vi "ni579x Configure Output Power.vi"(0 "Register Bus":T1, 1 "scope":string="tx", 5 "output power [dBm]":dbl, 9 "frequency [Hz]":dbl format="%#_6p", 11 "Error In":errorcluster, 12 "characterization data":T2 {"Frequencies [Hz]" format="%#_6p"}, 13 "correct IQ imbalance?":bool=TRUE) -> (4 "Register Bus (out)":T1, 6 "coerced output power [dBm]":dbl, 8 "digital gain":T6, 10 "IQ impairment correction":T5, 15 "Error Out":errorcluster)   [LabVIEW 2015, in "ni579x Config v2 Host.lvlib"]
doc: "Configures the Tx front end attenuators and filters to achieve the specified output power, returns the IQ impairment correction data which can be used to correct IQ impairments, and returns the residual digital gain that can be applied to the signal to achieve the specified output power. Also sets the RF filter appropriately for the specified frequency.\n\n<B>Input Parameters</B>\n\n<B>Register Bus</B> The Register Bus object created by the ni579x Open VI and used as the session handle for the NI-579x Configuration Design Library.\n\n<B>scope</B> Specifies which channel to configure. Can be \"tx\".\n\n<B>output power [dBm]</B> Specifies the power (in dBm) at the output terminal of the device that will correspond to the full-scale range of the DAC binary data.\n\n<B>frequency [Hz]</B> Specifies the frequency the LO is tuned to in the current configuration.\n\n<B>correct IQ imbalance?</B> Specifies whether this VI should calculate the IQ impairment correction values. Set to false if you are not using the IQ impairment correction DSP blocks in the FPGA.\n\n<B>characterization data</B> A set of data that describes the characteristics of this device that allows the VI to calculate the proper attenuation and IQ imbalance correction settings for the specified frequency. This data is stored in the EEPROM and can be retrieved using the ni579x Load Characterization Data (EEPROM) VI. For the 5791, the Tx data is index 1 in the array of characterization data returned by ni579x Load Characterization Data (EEPROM).vi\n\n<B>Output Parameters</B>\n\n<B>Register Bus (out)</B> The Register Bus object created by the ni579x Open VI and used as the session handle for the NI-579x Configuration Design Library.\n\n<B>coerced output power [dBm]</B> The actual output power the device was configured to (not including any additional digital gain applied by the DSP block in the FPGA... see the \"digital gain\" parameter for more information).\n\n<B>digital gain</B> There may be residual digital gain that needs to be applied to the data using the DSP blocks in the FPGA in order to achieve the requested output power. You can supply these residual gain values to the DSP Gain block in the FPGA.\n\n<B>IQ impairment correction</B> The values to apply to the IQ Impairment Correction DSP block in the FPGA, in order to correct gain and phase imbalances in the mixer."
uses:
  <instrlib>/ni579x/Config/v2/Host/ni579x Config v2 Host.lvlib
  <instrlib>/_niInstr/DSP/v1/Shared/Public/IQ Gain.ctl
  <instrlib>/_niInstr/DSP/v1/Shared/Public/IQ Impairments.ctl
  <instrlib>/ni579x/Config/v2/Shared/Types/ni579x Characterization Data.ctl
  <instrlib>/ni579x/Config/v2/Shared/Types/ni579x IQ Imbalance.ctl
  <instrlib>/ni579x/Config/v2/Shared/Types/ni579x Gain to Attenuation Mapping.ctl
  <instrlib>/_niInstr/Register Bus/v0/Host/Public/Register Bus Session.ctl
  <instrlib>/_niInstr/Register Bus/v0/Host/Private/Session Data.ctl
  <instrlib>/_niInstr/DSP/v1/Shared/niInstr DSP v1 Shared.lvlib
  <instrlib>/ni579x/Config/v2/Shared/ni579x Config v2 Shared.lvlib
  <instrlib>/_niInstr/Register Bus/v0/Host/niInstr Register Bus v0 Host.lvlib
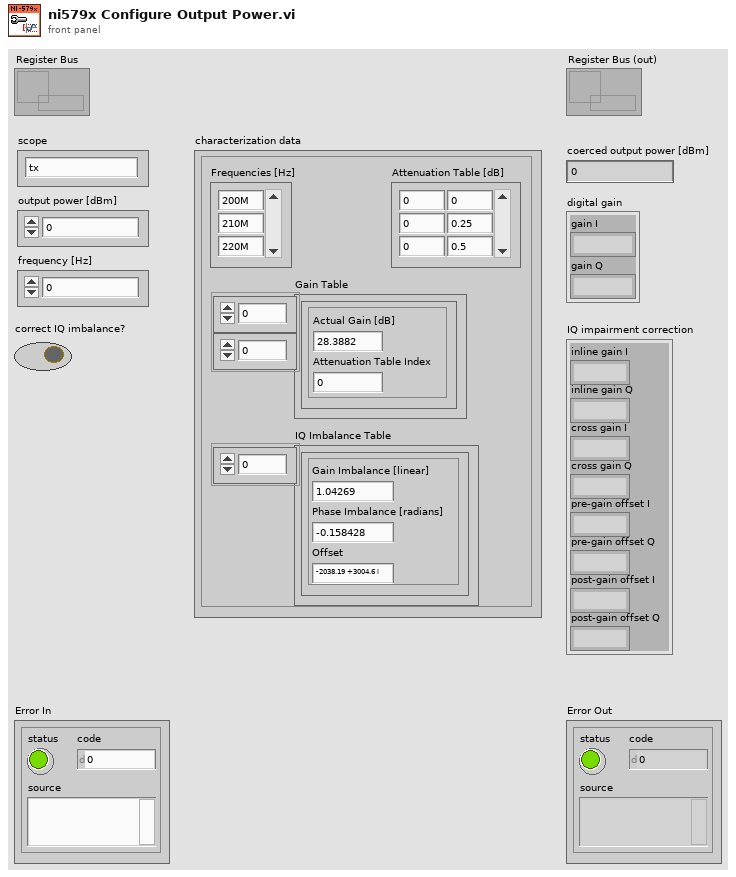
[diagram p1: front panel]
types:
  T1 = typedef "niInstr Register Bus v0 Host.lvlib/Register Bus Session.ctl" = refnum<queue>
  T2 = typedef "ni579x Config v2 Shared.lvlib/ni579x Characterization Data.ctl" = cluster{"Attenuation Table [dB]":dbl[][], "Frequencies [Hz]":dbl[], "IQ Imbalance Table":T3[], "Gain Table":T4[][]}
  T3 = typedef "ni579x Config v2 Shared.lvlib/ni579x IQ Imbalance.ctl" = cluster{"Gain Imbalance [linear]":dbl, "Phase Imbalance [radians]":dbl, "Offset":cdb}
  T4 = typedef "ni579x Config v2 Shared.lvlib/ni579x Gain to Attenuation Mapping.ctl" = cluster{"Actual Gain [dB]":dbl, "Attenuation Table Index":i32}
  T5 = typedef "niInstr DSP v1 Shared.lvlib/IQ Impairments.ctl" = cluster{"inline gain I":fxp<+/-,18,1>, "inline gain Q":fxp<+/-,18,1>, "cross gain I":fxp<+/-,18,1>, "cross gain Q":fxp<+/-,18,1>, "pre-gain offset I":fxp<+/-,18,1>, "pre-gain offset Q":fxp<+/-,18,1>, "post-gain offset I":fxp<+/-,18,1>, "post-gain offset Q":fxp<+/-,18,1>}
  T6 = typedef "niInstr DSP v1 Shared.lvlib/IQ Gain.ctl" = cluster{"gain I":fxp<+/-,24,3>, "gain Q":fxp<+/-,24,3>}
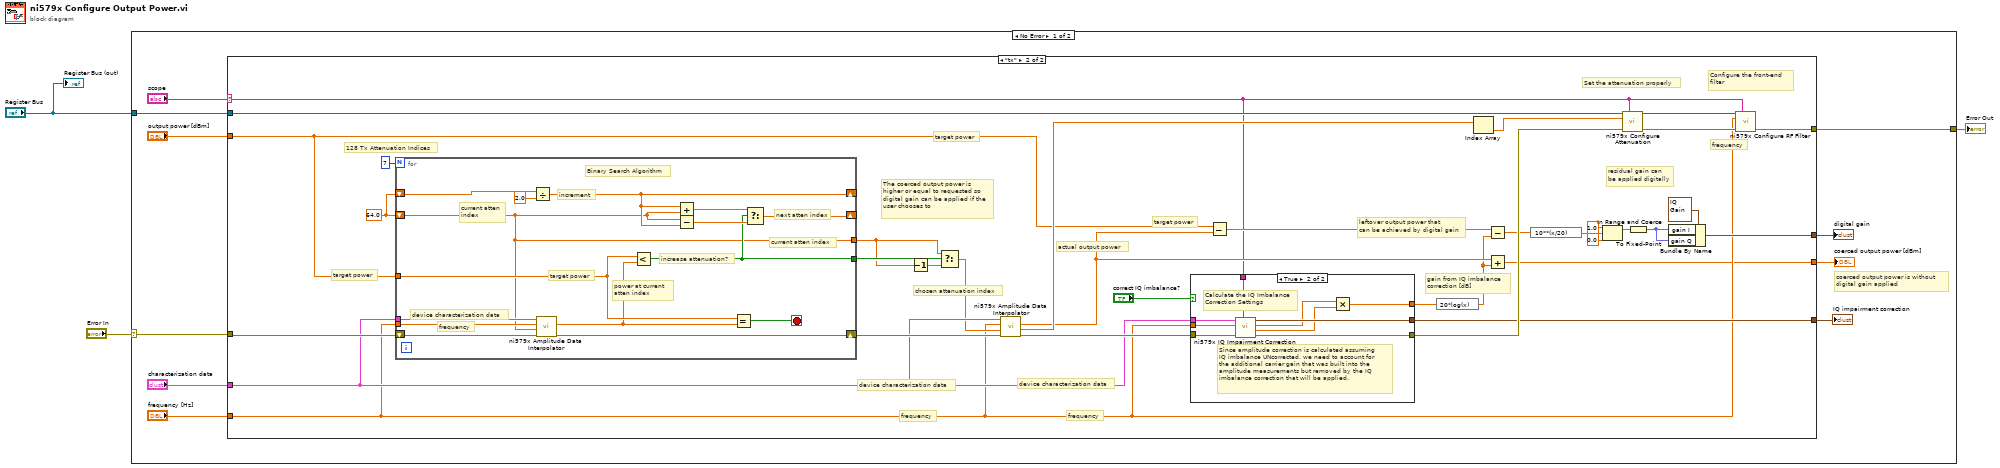
[diagram p0: block diagram]
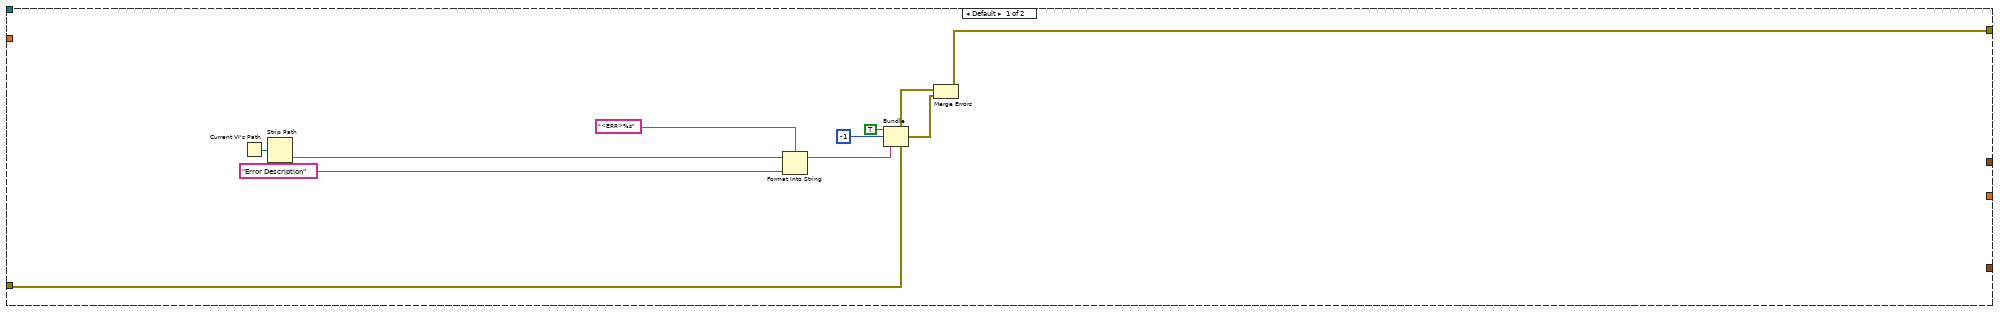
[diagram p2: hidden frame]
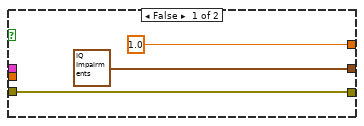
[diagram p3: hidden frame]
diagram:
  n1 = case shown="No Error" "Error In" {
    selector: "Error In" -> [w8 w86]
    tunnel: [w7 w86] -> w2
    tunnel: "Register Bus" -> [w9 _]
    frame No Error {
      # "coerced output power is without\ndigital gain applied"
      n2 = case shown="\"tx\"" "scope" {
        selector: "scope" -> [_ w31]
        tunnel: "output power [dBm]" -> [_ w38]
        tunnel: "frequency [Hz]" -> [_ w29]
        tunnel: "characterization data" -> [_ w39]
        tunnel: w9 -> [_ w58]
        tunnel: w8 -> [w15 w41]
        tunnel: [w14 w30] -> w7
        tunnel: [_ w56] -> w6
        tunnel: [_ w27] -> w5
        tunnel: [_ w49] -> w4
        frame Default {
          n3 = Current VI's Path() -> (path=w17:path)
          n4 = Strip Path(path=w17) -> (name=w18:string)  [unwired: 1 out]
          n5 = Format Into String(format string="<ERR>%s", initial string=w18, "Error Description" ("input 1")) -> (resulting string=w19:string)  [unwired: 1 in, 1 out]
          n6 = Bundle(cluster=w15, "status"=TRUE, "code"=-1, "source"=w19) -> (w20:errorcluster)
          n7 = Merge Errors(w15, w20) -> (w14:errorcluster)
        }
        frame "tx" {
          w43 = 64.0
          # "gain from IQ imbalance \ncorrection [dB]"
          # "leftover output power that \ncan be achieved by digital gain"
          # "frequency"
          # "Configure the front-end\nfilter"
          # "frequency"
          # "device characterization data"
          # "frequency"
          # "device characterization data"
          # "actual output power"
          # "target power"
          # "target power"
          # "residual gain can \nbe applied digitally"
          # "Set the attenuation properly"
          # "chosen attenuation index"
          # "target power"
          # "128 Tx Attenuation Indices"
          # "The coerced output power is\nhigher or equal to requested so \ndigital gain can be applied if the\nuser chooses to"
          n8 = for {
            N: 7 -> [_]
            tunnel: w39 -> [w75]
            tunnel: w29 -> [w74]
            tunnel: w38 -> [w76]
            shift-right: [w84] -> w40
            shift-left: w41 -> [w85]
            shift-right: [w78] -> _
            shift-left: w43 -> [w71]
            shift-right: [w77] -> _
            shift-left: w43 -> [w80]
            tunnel: [w71] -> w35
            tunnel: [w72] -> w36
            stop <- w83 stop-if-true
            # "device characterization data"
            # "frequency"
            # "target power"
            # "power at current \natten index"
            # "current atten index"
            # "next atten index"
            # "increase attenuation?"
            # "increment"
            # "current atten\nindex"
            # "Binary Search Algorithm"
            n9 = Divide(x=w80, y=2.0) -> (x/y=w77:dbl)
            n10 = call <instrlib>:"ni579x Amplitude Data Interpolator.vi"("Error In"=w85, "attenuation index"=w71, "frequency [Hz]"=w74, "characterization data"=w75) -> ("Error Out"=w84:errorcluster, "amplitude data"=w73:dbl)  [unwired: 5 in, 1 out]
            n11 = Less?(x=w76, y=w73) -> (x < y?=w72:bool)
            n12 = Add(x=w77, y=w71) -> (x+y=w82:dbl)
            n13 = Subtract(x=w71, y=w77) -> (x-y=w81:dbl)
            n14 = Equal?(x=w76, y=w73) -> (x = y?=w83:bool)
            n15 = Select(t=w82, s=w72, f=w81) -> (s? t:f=w78:dbl)
          }
          n16 = Decrement(x=w35) -> (x-1=w37:dbl)
          n17 = Select(t=w35, s=w36, f=w37) -> (s? t:f=w34:dbl)
          n18 = call <instrlib>:"ni579x Amplitude Data Interpolator.vi"("Error In"=w40, "attenuation index"=w34, "frequency [Hz]"=w29, "characterization data"=w39) -> ("Error Out"=w55:errorcluster, "attenuator values [dB]"=w54:dbl[], "amplitude data"=w50:dbl)  [unwired: 5 in]
          n19 = case shown="True" "correct IQ imbalance?" {
            tunnel: [w59 w70] -> w57
            tunnel: [T5 {"inline gain I"=0.9999923706054688, "inline gain Q"=0.9999923706054688, "cross gain I"=0.0, "cross gain Q"=0.0, "pre-gain offset I"=0.0, "pre-gain offset Q"=0.0, "post-gain offset I"=0.0, "post-gain offset Q"=0.0} ("IQ impairment") w69] -> w56
            tunnel: w55 -> [w59 w68]
            tunnel: w39 -> [_ w67]
            tunnel: w31 -> [_ w66]
            tunnel: w29 -> [_ w65]
            tunnel: [1.0 ("correction gain") w64] -> w26
            frame False {
            }
            frame True {
              # "Since amplitude correction is calculated assuming\nIQ imbalance UNcorrected, we need to account for\nthe additional carrier gain that was built into the\namplitude measurements but removed by the IQ\nimbalance correction that will be applied."
              # "Calculate the IQ Imbalance\nCorrection Settings"
              n20 = call <instrlib>:"ni579x IQ Impairment Correction.vi"("scope"=w66, "Error In"=w68, "frequency [Hz]"=w65, "characterization data"=w67) -> ("Error Out"=w70:errorcluster, "uncorrected carrier gain"=w62:dbl, "correction gain"=w63:dbl, "IQ impairment correction out"=w69:T5)  [unwired: 4 in]
              n21 = Multiply(x=w63, y=w62) -> (x*y=w64:dbl)
            }
          }
          n22 = Subtract(x=w38, y=w50) -> (x-y=w53:dbl)
          n23 = expression code="20*log(x)"(w26) -> (w25:dbl)
          n24 = Index Array(array=w54) -> (element=w44:dbl)  [unwired: 1 in]
          n25 = Subtract(x=w53, y=w25) -> (x-y=w28:dbl)
          n26 = Add(x=w50, y=w25) -> (x+y=w27:dbl)
          n27 = expression code="10**(x/20)"(w28) -> (w48:dbl)
          n28 = In Range and Coerce(upper limit=1.0, x=w48, lower limit=0.0) -> (coerced(x)=w46:dbl)  [unwired: 1 out]
          n29 = call <instrlib>:"ni579x Configure Attenuation.vi"("Register Bus"=w58, "scope"=w31, "attenuation [dB]"=w44, "Error In"=w57) -> ("Register Bus (out)"=w32:T1, "Error Out"=w33:errorcluster)  [unwired: 9 in, 1 out]
          n30 = To Fixed-Point(number=w46) -> (fixed-point=w51:fxp<+/-,24,3>)  [unwired: 1 in]
          n31 = Bundle By Name(cluster=T6 {"gain I"=0.9999923706054688, "gain Q"=0.9999923706054688} ("digital gain"), "gain I"=w51, "gain Q"=w51) -> (w49:T6)
          n32 = call <instrlib>:"ni579x Configure RF Filter.vi"("Register Bus"=w32, "scope"=w31, "frequency [Hz]"=w29, "Error In"=w33) -> ("Error Out"=w30:errorcluster)  [unwired: 9 in, 2 out]
        }
      }
      "IQ impairment correction" <- w6
      "digital gain" <- w4
      "coerced output power [dBm]" <- w5
    }
    frame Error {
    }
  }
  "Error Out" <- w2
  "Register Bus (out)" <- "Register Bus"
